vi "add set RP100 voltage.vi"(11 "字符串 2":string) -> (1 "ok or cancel":bool, 3 "连接的字符串 2":string)   [LabVIEW 2019, in "nematic.lvlib" / "Copy of StrainCell.lvlib"]
uses:
  nematic/Copy of StrainCell.lvlib
panel:
  in  "电压 (V) 2":dbl
  in  "cancel 2":bool
  in  "ok 2":bool
  in  "电压 (V)":dbl
  in  "slew (V/sec）":dbl=1.0
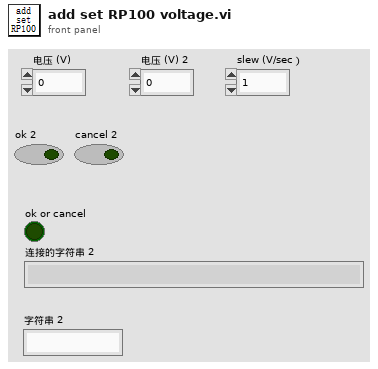
[diagram p1: front panel]
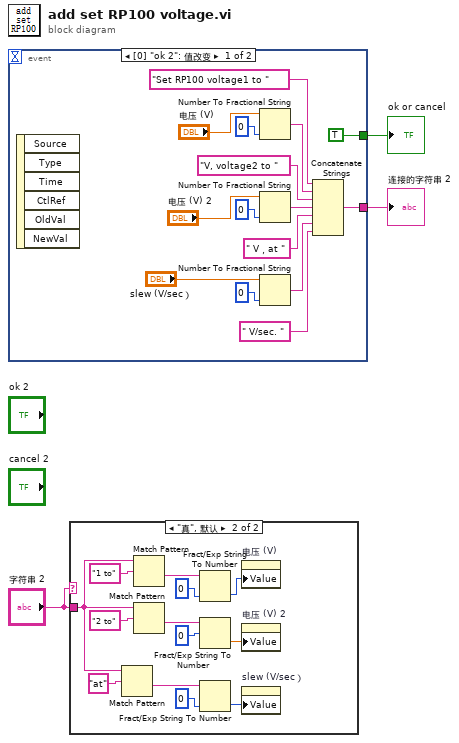
[diagram p0: block diagram]
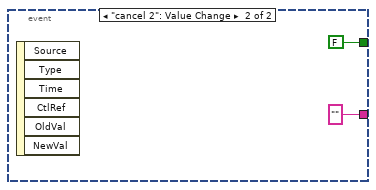
[diagram p3: hidden frame]
diagram:
  n1 = event shown="[0] \"ok 2\": 值改变" {
    selector: _ -> [_ _]
    dyn-events: _ -> [_ _]
    timeout: _ -> [_ _]
    tunnel: [TRUE FALSE] -> w2
    tunnel: [w10 "" ("分隔符")] -> w3
    event "ok 2": Value Change {
      n2 = event-data() -> ()  [unwired: 1 in, 6 out]
      n3 = Number To Fractional String(number="电压 (V)", precision (6)=i16 0 ("精度(6)")) -> (F-format string=w16:string)  [unwired: 2 in]
      n4 = Number To Fractional String(number="电压 (V) 2", precision (6)=i16 0 ("精度(6)")) -> (F-format string=w4:string)  [unwired: 2 in]
      n5 = Number To Fractional String(number="slew (V/sec）", precision (6)=i16 0 ("精度(6)")) -> (F-format string=w12:string)  [unwired: 2 in]
      n6 = Concatenate Strings("Set RP100 voltage1 to " ("字符串"), w16, "V, voltage2 to " ("string"), w4, " V，at " ("字符串"), w12, " V/sec. " ("字符串")) -> (w10:string)
    }
    event "cancel 2": Value Change {
      n7 = event-data() -> ()  [unwired: 1 in, 6 out]
    }
  }
  "ok or cancel" <- w2
  "连接的字符串 2" <- w3
  n8 = case shown="\"真\", 默认" "字符串 2" {
    tunnel: "字符串 2" -> [_ w25]
    frame "" {
    }
    frame "真", Default {
      n9 = Match Pattern(string=w25, regular expression="at" ("正则表达式")) -> (after substring=w28:string)  [unwired: 1 in, 3 out]
      n10 = Match Pattern(string=w25, regular expression="1 to" ("正则表达式")) -> (after substring=w31:string)  [unwired: 1 in, 3 out]
      n11 = Match Pattern(string=w25, regular expression="2 to" ("正则表达式")) -> (after substring=w23:string)  [unwired: 1 in, 3 out]
      n12 = Fract/Exp String To Number(string=w31, default (0 dbl)=0) -> (number=w27:i32)  [unwired: 2 in, 1 out]
      n13 = Fract/Exp String To Number(string=w23, offset=0) -> (number=w21:dbl)  [unwired: 2 in, 1 out]
      n14 = Fract/Exp String To Number(string=w28, default (0 dbl)=0) -> (number=w26:i32)  [unwired: 2 in, 1 out]
      n15 = property on="电压 (V)" class="DigNum (严格)"("Value"=w27) -> ()  [unwired: 2 in, 2 out]
      n16 = property on="电压 (V) 2" class="DigNum (严格)"("Value"=w21) -> ()  [unwired: 2 in, 2 out]
      n17 = property on="slew (V/sec）" class="DigNum (严格)"("Value"=w26) -> ()  [unwired: 2 in, 2 out]
    }
  }
